vi "WriteData.vi"(8 "error in (no error)":errorcluster, 10 "Value":dbl, 11 "reference in":refnum<class "Digital.lvclass">) -> (0 "error out":errorcluster, 3 "reference out":refnum<class "Digital.lvclass">)   [LabVIEW 2019, in "Digital.lvclass"]
uses:
  Digital.lvclass
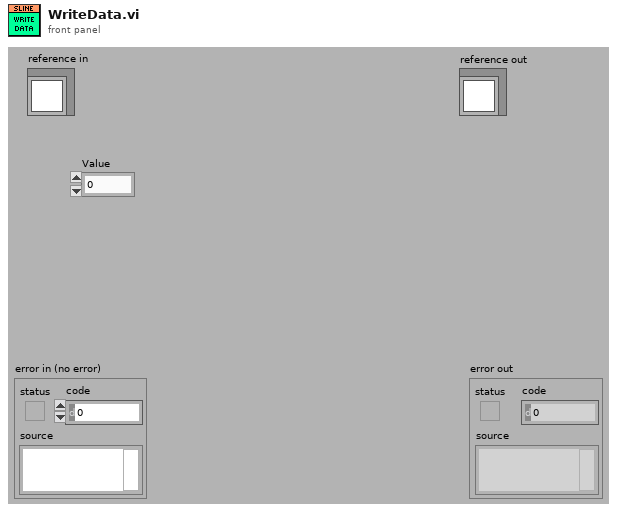
[diagram p1: front panel]
types:
  T1 = typedef "Digital.lvclass/ObjectAttributes.ctl" = cluster{"Override size":cluster{"Width":i16, "Height":i16}, "Value":dbl, "Digits Total":dbl, "Digits Precision":dbl}
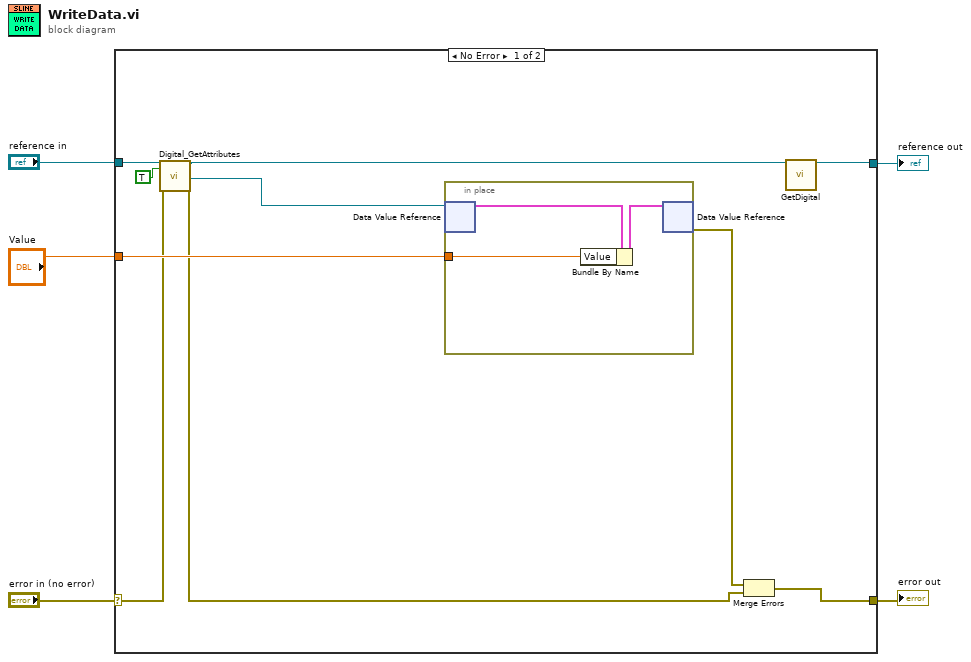
[diagram p0: block diagram]
diagram:
  n1 = case shown="No Error" "error in (no error)" {
    selector: "error in (no error)" -> [w9 w20]
    tunnel: [w13 w20] -> w4
    tunnel: [w6 w19] -> w2
    tunnel: "reference in" -> [w12 w19]
    tunnel: "Value" -> [w15 _]
    frame No Error {
      n2 = call "Digital_GetAttributes.vi"("reference in"=w12, "OnlyGetDvrReference(False)"=TRUE, "error in (no error)"=w9) -> ("reference out"=w11:refnum<class "Digital.lvclass">, "DataRef"=w10:refnum<data-value>, "error out"=w8:errorcluster)  [unwired: 13 in, 1 out]
      n3 = in-place {
        in-place-border: w15 -> [w18]
        n4 = in-place-dvr #1(w10) -> (w17:T1)  [unwired: 1 out]
        n5 = Bundle By Name(cluster=w17, "Value"=w18) -> (w16:T1)
        n6 = in-place-dvr #1(w16) -> (w14:errorcluster)  [unwired: 1 out]
      }
      n7 = Merge Errors(w14, w8) -> (w13:errorcluster)
      n8 = call-dynamic "GetDigital.vi"("reference in"=w11) -> ("reference out"=w6:refnum<class "Digital.lvclass">)  [unwired: 17 in, 1 out]
    }
    frame Error {
    }
  }
  "error out" <- w4
  "reference out" <- w2
